vi "Actor Core.vi"(8 "error in":errorcluster, 11 "Measure Object in":refnum<class "Sequence Element.lvclass">) -> (0 "error out":errorcluster, 3 "Actor out":refnum<class "Actor.lvclass">)   [LabVIEW 2016, in "Sequence Element.lvclass"]
doc: "(<B>Filename</B>: Actor Framework.lvlib:Actor.lvclass:Actor Core.vi)\n\nReceives messages to the actor, reacts to them, and initiates any error handling that may shut the actor down.\n\nDescendant classes may override this VI to append parallel tasks for the actor to complete while it handles messages. Overrides use the Call Parent Method node."
uses:
  Sequence Element.lvclass
  C:/github/LabActor/Template Module/Template Module.lvclass
  C:/Program Files/National Instruments/LabVIEW 2016/vi.lib/ActorFramework/Actor/Actor.lvclass
  <vilib>/ActorFramework/Actor/Actor.lvclass
  Sequence Element.lvclass/Sequence Element.ctl
  Template Module/Template Module.lvclass/Template Module.ctl
  <vilib>/ActorFramework/Actor/Actor.lvclass/Actor.ctl
  <vilib>/ActorFramework/Message Enqueuer/Message Enqueuer.lvclass/Message Enqueuer.ctl
  Sequence Element Messages/Items Mouse Click Msg/Items Mouse Click Msg.lvclass/Items Mouse Click Msg.ctl
  Template Module/Read stop event.vi
  <vilib>/ActorFramework/Message Enqueuer/Init from Existing Queue.vi
  <vilib>/ActorFramework/Message Enqueuer/Enqueue.vi
  Template Module Messages/Configuration Value Changed Msg/Configuration Value Changed Msg.lvclass
  C:/Program Files/National Instruments/LabVIEW 2016/vi.lib/ActorFramework/Message/Message.lvclass
  Sequence Element Messages/Items Mouse Click Msg/Items Mouse Click Msg.lvclass
  <vilib>/ActorFramework/Message Priority Queue/Priority Enqueue.vi
  Worker/Worker.lvclass
  <vilib>/ActorFramework/Message Enqueuer/Message Enqueuer.lvclass
panel:
  out "Name":string
  in  "Configuration":T1={"Start"=0.0, "End"=1.0, "Duration"=60.0, "Instrument"=-1} {"Duration" format="%#_6ps"}
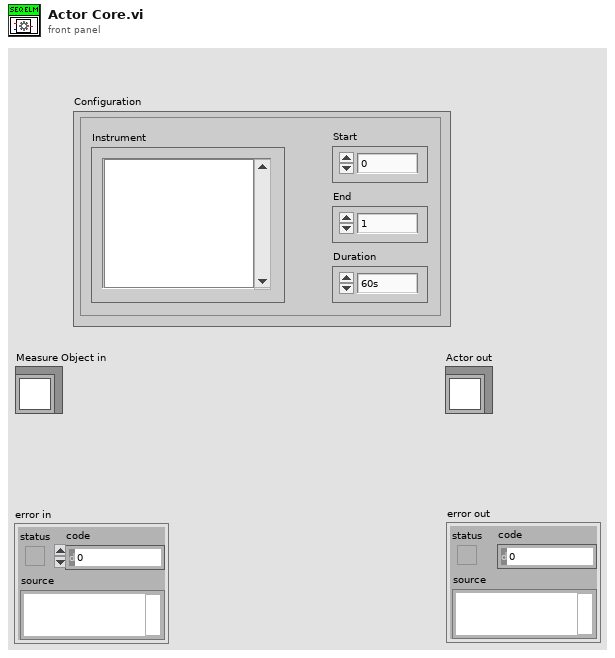
[diagram p1: front panel]
types:
  T1 = cluster{"Start":dbl, "End":dbl, "Duration":dbl, "Instrument":i32}
  T2 = typedef "LVPoint32TypeDef.ctl" = cluster{"Horizontal":i32, "Vertical":i32}
  T3 = cluster{"Shift":bool, "Ctrl":bool, "Alt":bool, "Cmd":bool, "Opt":bool}
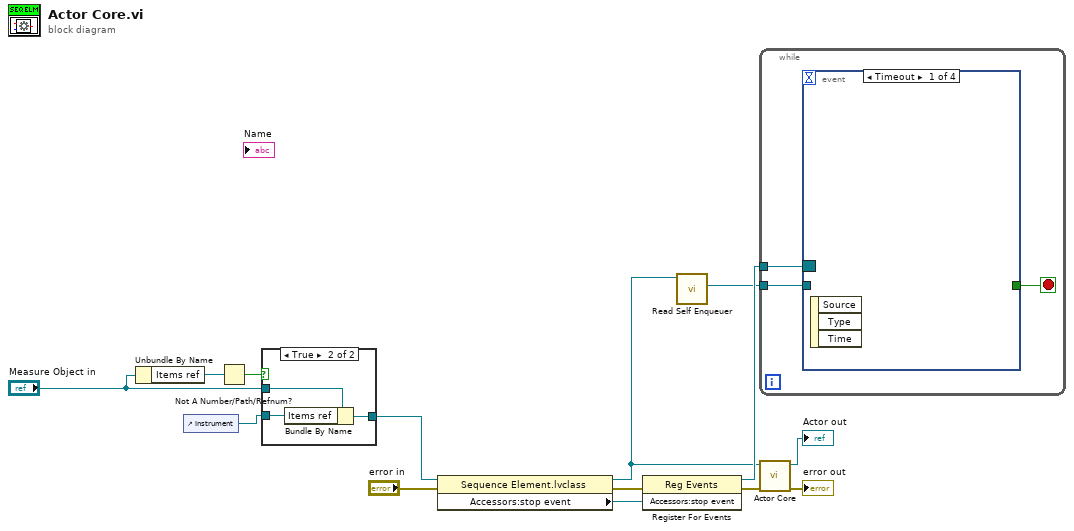
[diagram p0: block diagram]
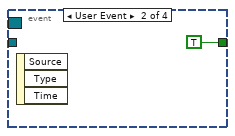
[diagram p3: hidden frame]
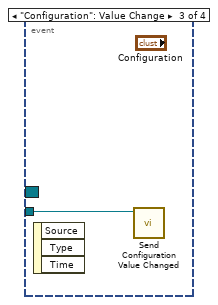
[diagram p4: hidden frame]
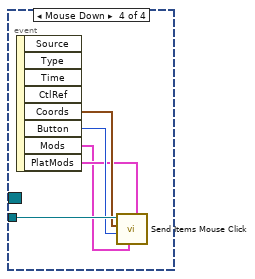
[diagram p5: hidden frame]
diagram:
  n1 = Unbundle By Name("Measure Object in") -> ("Items ref"=w2:refnum<vi>)
  n2 = control-ref of="Instrument"() -> (w4:refnum<vi>)
  n3 = Not A Number/Path/Refnum?(number/path/refnum=w2) -> (NaN/Path/Refnum?=w1:bool)
  n4 = case shown="True" w1 {
    tunnel: [w15 w18] -> w5
    tunnel: w4 -> [_ w17]
    tunnel: "Measure Object in" -> [w15 w16]
    frame False {
    }
    frame True {
      n5 = Bundle By Name(cluster=w16, "Items ref"=w17) -> (w18:refnum<class "Sequence Element.lvclass">)
    }
  }
  n6 = property class="Sequence Element.lvclass"(reference=w5, error in="error in") -> (reference out=w8:refnum<class "Sequence Element.lvclass">, error out=w12:errorcluster, "Accessors:stop event"=w11:refnum<user-event>)
  n7 = register-events(error in=w12, w11) -> (reference out=w10:refnum<event-registration>, error out=w6:errorcluster)  [unwired: 1 in]
  n8 = call <vilib>:"Read Self Enqueuer.vi"("Actor"=w8) -> ("Self Enqueuer"=w9:refnum<class "Message Enqueuer.lvclass">)  [unwired: 10 in]
  n9 = while {
    tunnel: w10 -> [w21]
    tunnel: w9 -> [w19]
    stop <- w20 stop-if-true
    n10 = event shown="[0] Timeout" {
      selector: w21 -> [_ _ _ _]
      dyn-events: _ -> [_ _ _ _]
      timeout: _ -> [_ _ _ _]
      tunnel: [_ TRUE _ _] -> w20
      tunnel: w19 -> [_ _ w23 w28]
      event Timeout {
        n11 = event-data() -> ()  [unwired: 1 in, 3 out]
      }
      event User Event {
        n12 = event-data() -> ()  [unwired: 1 in, 3 out]
      }
      event "Configuration": Value Change {
        n13 = event-data() -> ()  [unwired: 1 in, 3 out]
        n14 = call "Send Configuration Value Changed.vi"("Message Enqueuer"=w23) -> ()  [unwired: 9 in, 2 out]
      }
      event "Configuration.Instrument": Mouse Down {
        n15 = event-data() -> ("Coords"=w27:T2, "Button"=w26:u16, "Mods"=w24:cluster{"Double Click":bool, "Menu Key":bool}, "PlatMods"=w25:T3)  [unwired: 1 in, 4 out]
        n16 = call "Send Items Mouse Click.vi"("PlatMods"=w25, "Mods"=w24, "Button"=w26, "Coords"=w27, "Message Enqueuer"=w28) -> ()  [unwired: 5 in, 2 out]
      }
    }
  }
  n17 = call-parent "Actor Core.vi"("error in"=w6, "Measure Object in"=w8) -> ("error out"=→"error out":errorcluster, "Actor out"=→"Actor out":refnum<class "Actor.lvclass">)  [unwired: 8 in]
